vi "receive_01normal.vi"() -> ()   [LabVIEW 2015]
uses:
  <instrlib>/niUSRP/niUSRP Fetch Rx Data (CDB Cluster).vi
  <vilib>/addons/Modulation/Analog/MT Demodulate AM (DSB).vi
  <vilib>/addons/Modulation/niAMT.lvlib
panel:
  out "Meta Information:Driver Identification:Current Driver Version":string
  in  "modulation index":dbl=1.0 format="%.2f"
  out "AM demodulated":waveform(dbl)(graph)
  in  "active antenna":string="RX2"
  in  "Channels":string(combo)="0"
  out "Waveform Magnitude":cluster{"t0":dbl, "dt":dbl, "Y":dbl[]}(graph)
  in  "Stop":bool
  out "coerced gain":dbl format="%#_6f"
  out "coerced carrier frequency":dbl=100000.0 format="%#_6p"
  out "coerced IQ rate":dbl=100000.0 format="%#_6p"
  in  "gain":dbl format="%#_6f"
  in  "carrier frequency":dbl=920000000.0 format="%#_6p"
  in  "IQ rate":dbl=2000000.0 format="%#_6p"
  in  "number of samples":i64=2000000
  in  "timeout":dbl=10.0
  out "error out":errorcluster
  in  "device names":refnum<k15>="192.168.10.14"
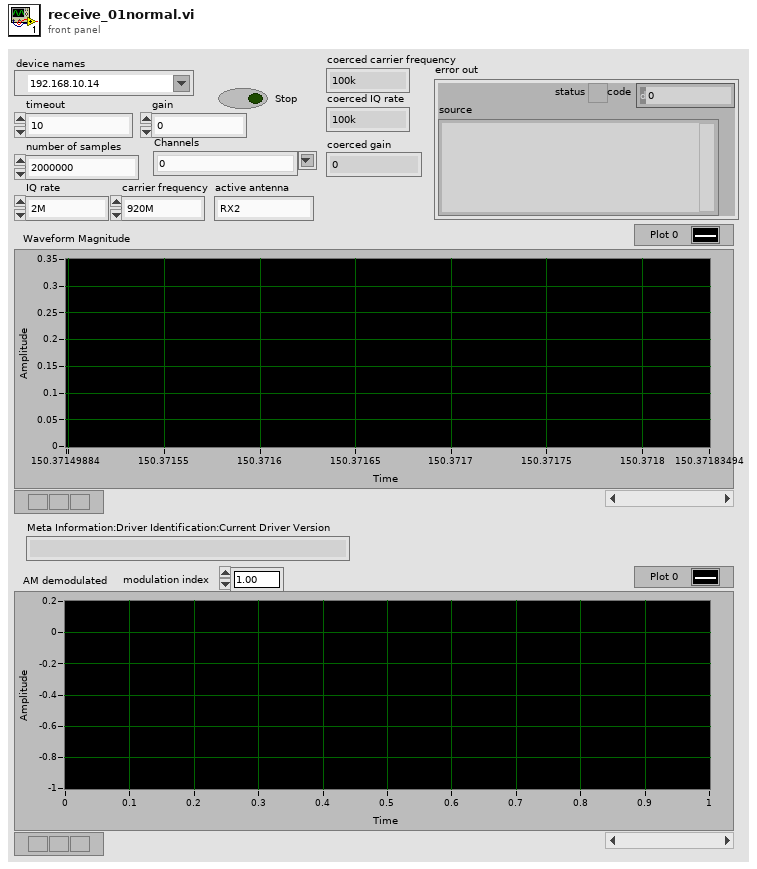
[diagram p1: front panel]
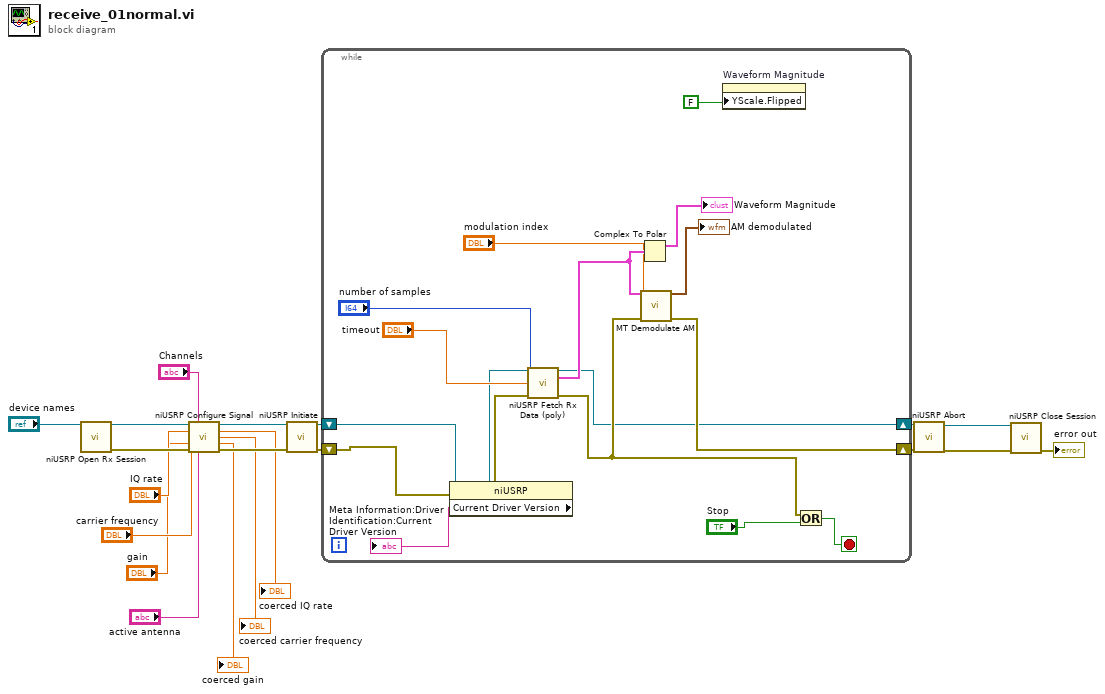
[diagram p0: block diagram]
diagram:
  n1 = call <instrlib>:"niUSRP Open Rx Session.vi"("device names"="device names") -> ("session handle out"=w19:refnum<k15>, "error out"=w18:errorcluster)  [unwired: 13 in]
  n2 = call <instrlib>:"niUSRP Configure Signal.vi"("session handle"=w19, "channel list"="Channels", "IQ rate"="IQ rate", "carrier frequency"="carrier frequency", "gain"="gain", "error in (no error)"=w18, "active antenna"="active antenna") -> ("session handle out"=w17:refnum<k15>, "coerced IQ rate"=→"coerced IQ rate":dbl, "coerced carrier frequency"=→"coerced carrier frequency":dbl, "coerced gain"=→"coerced gain":dbl, "error out"=w16:errorcluster)  [unwired: 4 in]
  n3 = call <instrlib>:"niUSRP Initiate.vi"("session handle"=w17, "error in (no error)"=w16) -> ("session handle out"=w15:refnum<k15>, "error out"=w14:errorcluster)  [unwired: 12 in]
  n4 = while {
    shift-right: [w26] -> w13
    shift-left: w15 -> [w25]
    shift-right: [w30] -> w12
    shift-left: w14 -> [w23]
    stop <- w35 stop-if-true
    n5 = property on="Property Node" class="niUSRP"(reference=w25, error in=w23) -> (reference out=w24:refnum<k15>, error out=w22:errorcluster, "Current Driver Version"=→"Meta Information:Driver Identification:Current Driver Version":string)
    n6 = call-poly <instrlib>:"niUSRP Fetch Rx Data (poly).vi"("session handle"=w24, "number of samples"="number of samples", "timeout"="timeout", "error in (no error)"=w22) -> ("session handle out"=w26:refnum<k15>, "data"=w32:cluster{"t0":dbl, "dt":dbl, "Y":cdb[]}, "error out"=w31:errorcluster)  [unwired: 8 in, 1 out]
    n7 = Complex To Polar(r * e^(i*theta)=w32) -> (r=→"Waveform Magnitude":cluster{"t0":dbl, "dt":dbl, "Y":dbl[]})  [unwired: 1 out]
    n8 = call-poly <vilib>:"MT Demodulate AM.vi"("AM modulated waveform"=w32, "modulation index"="modulation index", "error in (no error)"=w31) -> ("AM demodulated waveform"=→"AM demodulated":waveform(dbl), "error out"=w30:errorcluster)  [unwired: 10 in, 1 out]
    n9 = property on="Waveform Magnitude" class="WFGraph (strict)"("YScale.Flipped"=FALSE ("Y Scale.Flipped")) -> ()  [unwired: 2 in, 2 out]
    n10 = Or(x=w31, y="Stop") -> (x .or. y?=w35:bool)
  }
  n11 = call <instrlib>:"niUSRP Abort.vi"("session handle"=w13, "error in (no error)"=w12) -> ("session handle out"=w11:refnum<k15>, "error out"=w10:errorcluster)  [unwired: 12 in]
  n12 = call <instrlib>:"niUSRP Close Session.vi"("session handle"=w11, "error in (no error)"=w10) -> ("error out"=→"error out":errorcluster)  [unwired: 13 in]
